vi "Ignite plasma and sample diode readings v2.vi"() -> ()   [LabVIEW 2018]
uses:
  <vilib>/DAQmx/write.llb/DAQmx Write (Analog DBL 1Chan 1Samp).vi
  749e0d07-3b49-41a5-821b-d06d1e37d043.vi
  <vilib>/DAQmx/read.llb/DAQmx Read (Analog DBL 1Chan 1Samp).vi
  83b8862b-d51e-48d4-833c-e6335a73f844.vi
  <vilib>/DAQmx/create/channels.llb/DAQmx Create Channel (AI-Voltage-Basic).vi
  <vilib>/DAQmx/create/channels.llb/DAQmx Create Channel (AO-Voltage-Basic).vi
  <vilib>/DAQmx/miscellaneous.llb/DAQmx Fill In Error Info.vi
panel:
  in  "germanium":path=path "C:/Users/severinm/Desktop/germaniam diode - plasma on.lvm" caption="Filename"
  in  "polarimeter":path=path "C:/Users/severinm/Desktop/other diode - plasma on.lvm" caption="Filename"
  in  "Polarimeter":tag
  in  "stop":bool
  in  "Germanium Diode":tag
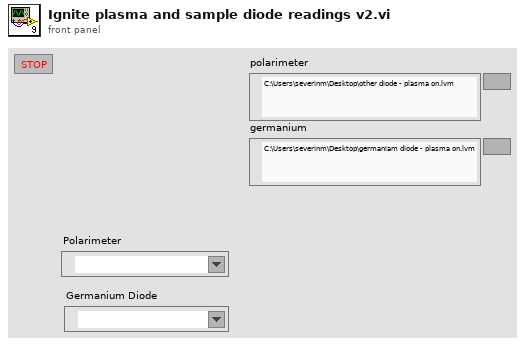
[diagram p1: front panel]
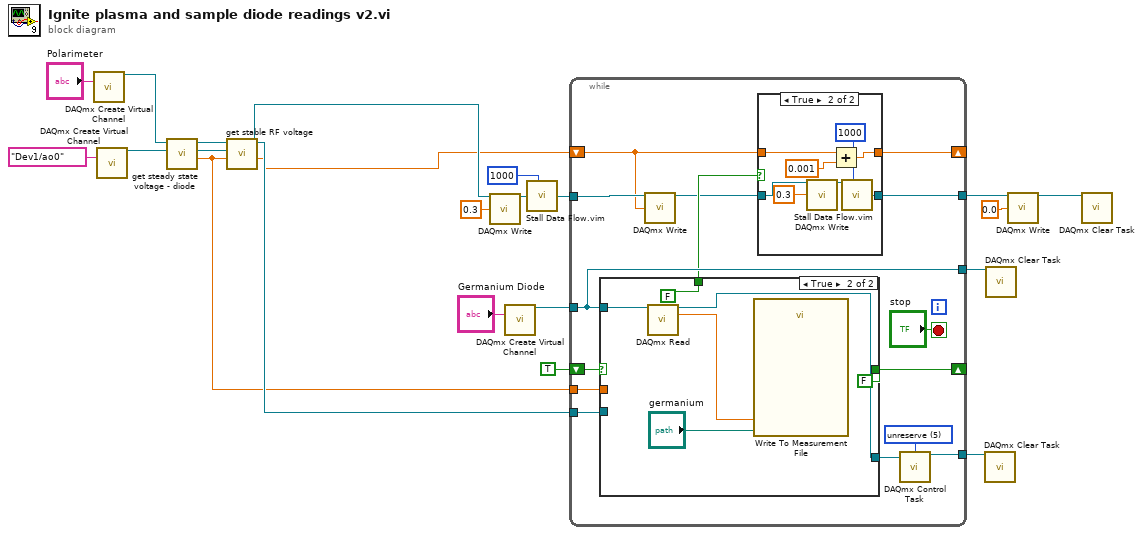
[diagram p0: block diagram]
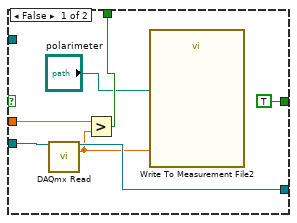
[diagram p3: hidden frame]
diagram:
  n1 = call-poly <vilib>:"DAQmx Create Virtual Channel.vi"("physical channels"="Polarimeter") -> ("task out"=w14:refnum<k21>)  [unwired: 13 in, 1 out]
  n2 = call-poly <vilib>:"DAQmx Create Virtual Channel.vi"("physical channels"=tag "Dev1/ao0") -> ("task out"=w13:refnum<k21>)  [unwired: 13 in, 1 out]
  n3 = call "get steady state voltage - diode.vi"("RF Generator Task In"=w13, "Diode Task In"=w14) -> ("Output"=w1:dbl, "RF Generator task out"=w5:refnum<k21>, "Diode task out"=w6:refnum<k21>)  [unwired: 7 in]
  n4 = call "get stable RF voltage.vi"("diode steady state voltage"=w1, "RF Generator task in"=w5, "Diode Task In"=w6) -> ("stable voltage"=w2:dbl, "RF generator task out"=w4:refnum<k21>, "diode task out"=w3:refnum<k21>)  [unwired: 6 in]
  n5 = call-poly <vilib>:"DAQmx Write.vi"("task/channels in"=w4, "data"=0.3) -> ("task out"=w12:refnum<k21>)  [unwired: 11 in, 2 out]
  n6 = call-poly <vilib>:"DAQmx Create Virtual Channel.vi"("physical channels"="Germanium Diode") -> ("task out"=w21:refnum<k21>)  [unwired: 13 in, 1 out]
  n7 = call "Stall Data Flow.vim"("value in"=w12, "milliseconds to wait"=u32 1000) -> ("value out"=w9:refnum<k21>)  [unwired: 1 out]
  n8 = while {
    tunnel: w21 -> [w34]
    shift-right: [w36] -> _
    shift-left: TRUE -> [w35]
    tunnel: [w34] -> w18
    tunnel: w3 -> [w31]
    tunnel: w9 -> [w30]
    shift-right: [w27] -> _
    shift-left: w2 -> [w28]
    tunnel: [w24] -> w8
    tunnel: [w26] -> w7
    tunnel: w1 -> [w23]
    stop <- "stop" stop-if-true
    w32 = 5 items=["verify"=2, "reserve"=4, "commit"=3, "unreserve"=5, "abort"=6] ("action")
    n9 = case shown="True" w35 {
      tunnel: w34 -> [_ w60]
      tunnel: [TRUE FALSE] -> w36
      tunnel: [w53 w57] -> w33
      tunnel: w31 -> [w52 _]
      tunnel: [w50 FALSE] -> w29
      tunnel: w23 -> [w48 _]
      frame False {
        n10 = call-poly <vilib>:"DAQmx Read.vi"("task/channels in"=w52) -> ("task out"=w53:refnum<k21>, "data"=w51:dbl)  [unwired: 12 in, 1 out]
        n11 = Greater?(x=w48, y=w51) -> (0:w50:bool)
        n12 = call "Write To Measurement File2"("Signals"=w51, "Filename"="polarimeter") -> ()  [unwired: 15 in, 3 out]
      }
      frame True {
        n13 = call-poly <vilib>:"DAQmx Read.vi"("task/channels in"=w60) -> ("task out"=w57:refnum<k21>, "data"=w59:dbl)  [unwired: 12 in, 1 out]
        n14 = call "Write To Measurement File"("Signals"=w59, "Filename"="germanium") -> ()  [unwired: 15 in, 3 out]
      }
    }
    n15 = call-poly <vilib>:"DAQmx Write.vi"("task/channels in"=w30, "data"=w28) -> ("task out"=w25:refnum<k21>)  [unwired: 11 in, 2 out]
    n16 = case shown="True" w29 {
      tunnel: w28 -> [w39 w47]
      tunnel: [w39 w45] -> w27
      tunnel: w25 -> [w38 w44]
      tunnel: [w38 w41] -> w24
      frame False {
      }
      frame True {
        n17 = call-poly <vilib>:"DAQmx Write.vi"("task/channels in"=w44, "data"=0.3) -> ("task out"=w43:refnum<k21>)  [unwired: 11 in, 2 out]
        n18 = Add(x=w47, y=0.001) -> (x+y=w45:dbl)
        n19 = call "Stall Data Flow.vim"("value in"=w43, "milliseconds to wait"=u32 1000) -> ("value out"=w41:refnum<k21>)  [unwired: 1 out]
      }
    }
    n20 = call <vilib>:"DAQmx Control Task.vi"("task/channels in"=w33, "action"=w32) -> ("task out"=w26:refnum<k21>)  [unwired: 12 in, 1 out]
  }
  n21 = call <vilib>:"DAQmx Clear Task.vi"("task in"=w7) -> ()  [unwired: 14 in, 1 out]
  n22 = call <vilib>:"DAQmx Clear Task.vi"("task in"=w18) -> ()  [unwired: 14 in, 1 out]
  n23 = call-poly <vilib>:"DAQmx Write.vi"("task/channels in"=w8, "data"=0.0) -> ("task out"=w15:refnum<k21>)  [unwired: 11 in, 2 out]
  n24 = call <vilib>:"DAQmx Clear Task.vi"("task in"=w15) -> ()  [unwired: 14 in, 1 out]
